vi "Format CSV.vi"(8 "error in (no error)":errorcluster, 9 "delimiter":string=",", 10 "CSV File Input":path, 11 "Original CSV Format":enum16{"Format A", "Format B"}(ring)) -> (0 "error out":errorcluster, 1 "Parcel Length":i32[](array[numeric]), 2 "All Terminal Data":T1(array[cluster]))   [LabVIEW 2017] (continued)
"40:47.0", "40:47.1", "40:47.1", "40:47.1", "40:47.2", "40:47.2", "40:47.2", "40:47.3", "40:47.3", "40:47.3", "40:47.4", "40:47.4", "40:47.4", "40:47.5", "40:47.5", "40:47.5", "40:47.6", "40:47.6", "40:47.6", "40:47.7", "40:47.7", "40:47.7", "40:47.8", "40:47.8", "40:47.8", "40:47.9", "40:47.9", "40:47.9", "40:48.0", "40:48.0", "40:48.0", "40:48.1", "40:48.1", "40:48.1", "40:48.2", "40:48.2", "40:48.2", "40:48.3", "40:48.3", "40:48.3", "40:48.4", "40:48.4", "40:48.4", "40:48.5", "40:48.5", "40:48.5", "40:48.6", "40:48.6", "40:48.6", "40:48.7", "40:48.7", "40:48.7", "40:48.8", "40:48.8", "40:48.8", "40:48.9", "40:48.9", "40:48.9", "40:49.0", "40:49.0", "40:49.0", "40:49.1", "40:49.1", "40:49.1", "40:49.2", "40:49.2", "40:49.2", "40:49.3", "40:49.3", "40:49.3", "40:49.4", "40:49.4", "40:49.4", "40:49.5", "40:49.5", "40:49.5", "40:49.6", "40:49.6", "40:49.6", "40:49.7", "40:49.7", "40:49.7", "40:49.8", "40:49.8", "40:49.8", "40:49.9", "40:49.9", "40:49.9", "40:50.0", "40:50.0", "40:50.0", "40:50.1", "40:50.1", "40:50.1", "40:50.2", "40:50.2", "40:50.2", "40:50.3", "40:50.3", "40:50.3", "40:50.4", "40:50.4", "40:50.4", "40:50.5", "40:50.5", "40:50.5", "40:50.6", "40:50.6", "40:50.6", "40:50.7", "40:50.7", "40:50.7", "40:50.8", "40:50.8", "40:50.8", "40:50.9", "40:50.9", "40:50.9", "40:51.0", "40:51.0", "40:51.0", "40:51.1", "40:51.1", "40:51.1", "40:51.2", "40:51.2", "40:51.2", "40:51.3", "40:51.3", "40:51.3", "40:51.4", "40:51.4", "40:51.4", "40:51.5", "40:51.5", "40:51.5", "40:51.6", "40:51.6", "40:51.6", "40:51.7", "40:51.7", "40:51.7", "40:51.8", "40:51.8", "40:51.8", "40:51.9", "40:51.9", "40:51.9", "40:52.0", "40:52.0", "40:52.0", "40:52.1", "40:52.1", "40:52.1", "40:52.2", "40:52.2", "40:52.2", "40:52.3", "40:52.3", "40:52.3", "40:52.4", "40:52.4", "40:52.4", "40:52.5", "40:52.5", "40:52.5", "40:52.6", "40:52.6", "40:52.6", "40:52.7", "40:52.7", "40:52.7", "40:52.8", "40:52.8", "40:52.8", "40:52.9", "40:52.9", "40:52.9", "40:53.0", "40:53.0", "40:53.0", "40:53.1", "40:53.1", "40:53.1", "40:53.2", "40:53.2", "40:53.2", "40:53.3", "40:53.3", "40:53.3", "40:53.4", "40:53.4", "40:53.4", "40:53.5", "40:53.5", "40:53.5", "40:53.6", "40:53.6", "40:53.6", "40:53.7", "40:53.7", "40:53.7", "40:53.8", "40:53.8", "40:53.8", "40:53.9", "40:53.9", "40:53.9", "40:54.0", "40:54.0", "40:54.0", "40:54.1", "40:54.1", "40:54.1", "40:54.2", "40:54.2", "40:54.2", "40:54.3", "40:54.3", "40:54.3", "40:54.4", "40:54.4", "40:54.4", "40:54.5", "40:54.5", "40:54.5", "40:54.6", "40:54.6", "40:54.6", "40:54.7", "40:54.7", "40:54.7", "40:54.8", "40:54.8", "40:54.8", "40:54.9", "40:54.9", "40:54.9", "40:55.0", "40:55.0", "40:55.0", "40:55.1", "40:55.1", "40:55.1", "40:55.2", "40:55.2", "40:55.2", "40:55.3", "40:55.3", "40:55.3", "40:55.4", "40:55.4", "40:55.4", "40:55.5", "40:55.5", "40:55.5", "40:55.6", "40:55.6", "40:55.6", "40:55.7", "40:55.7", "40:55.7", "40:55.8", "40:55.8", "40:55.8", "40:55.9", "40:55.9", "40:55.9", "40:56.0", "40:56.0", "40:56.0", "40:56.1", "40:56.1", "40:56.1", "40:56.2", "40:56.2", "40:56.2", "40:56.3", "40:56.3", "40:56.3", "40:56.4", "40:56.4", "40:56.4", "40:56.5", "40:56.5", "40:56.5", "40:56.6", "40:56.6", "40:56.6", "40:56.7", "40:56.7", "40:56.7", "40:56.8", "40:56.8", "40:56.8", "40:56.9", "40:56.9", "40:56.9", "40:57.0", "40:57.0", "40:57.0", "40:57.1", "40:57.1", "40:57.1", "40:57.2", "40:57.2", "40:57.2", "40:57.3", "40:57.3", "40:57.3", "40:57.4", "40:57.4", "40:57.4", "40:57.5", "40:57.5", "40:57.5", "40:57.6", "40:57.6", "40:57.6", "40:57.7", "40:57.7", "40:57.7", "40:57.8", "40:57.8", "40:57.8", "40:57.9", "40:57.9", "40:57.9", "40:58.0", "40:58.0", "40:58.0", "40:58.1", "40:58.1", "40:58.1", "40:58.2", "40:58.2", "40:58.2", "40:58.3", "40:58.3", "40:58.3", "40:58.4", "40:58.4", "40:58.4", "40:58.5", "40:58.5", "40:58.5", "40:58.6", "40:58.6", "40:58.6", "40:58.7", "40:58.7", "40:58.7", "40:58.8", "40:58.8", "40:58.8", "40:58.9", "40:58.9", "40:58.9", "40:59.0", "40:59.0", "40:59.0", "40:59.1", "40:59.1", "40:59.1", "40:59.2", "40:59.2", "40:59.2", "40:59.3", "40:59.3", "40:59.3", "40:59.4", "40:59.4", "40:59.4", "40:59.5", "40:59.5", "40:59.5", "40:59.6", "40:59.6", "40:59.6", "40:59.7", "40:59.7", "40:59.7", "40:59.8", "40:59.8", "40:59.8", "40:59.9", "40:59.9", "40:59.9", "41:00.0", "41:00.0", "41:00.0", "41:00.1", "41:00.1", "41:00.1", "41:00.2", "41:00.2", "41:00.2", "41:00.3", "41:00.3", "41:00.3", "41:00.4", "41:00.4", "41:00.4", "41:00.5", "41:00.5", "41:00.5", "41:00.6", "41:00.6", "41:00.6", "41:00.7", "41:00.7", "41:00.7", "41:00.8", "41:00.8", "41:00.8", "41:00.9", "41:00.9", "41:00.9", "41:01.0", "41:01.0", "41:01.0", "41:01.1", "41:01.1", "41:01.1", "41:01.2", "41:01.2", "41:01.2", "41:01.3", "41:01.3", "41:01.3", "41:01.4", "41:01.4", "41:01.4", "41:01.5", "41:01.5", "41:01.5", "41:01.6", "41:01.6", "41:01.6", "41:01.7", "41:01.7", "41:01.7", "41:01.8", "41:01.8", "41:01.8", "41:01.9", "41:01.9", "41:01.9", "41:02.0", "41:02.0", "41:02.0", "41:02.1", "41:02.1", "41:02.1", "41:02.2", "41:02.2", "41:02.2", "41:02.3", "41:02.3", "41:02.3", "41:02.4", "41:02.4", "41:02.4", "41:02.5", "41:02.5", "41:02.5", "41:02.6", "41:02.6", "41:02.6", "41:02.7", "41:02.7", "41:02.7", "41:02.8", "41:02.8", "41:02.8", "41:02.9", "41:02.9", "41:02.9", "41:03.0", "41:03.0", "41:03.0", "41:03.1", "41:03.1", "41:03.1", "41:03.2", "41:03.2", "41:03.2", "41:03.3", "41:03.3", "41:03.3", "41:03.4", "41:03.4", "41:03.4", "41:03.5", "41:03.5", "41:03.5", "41:03.6", "41:03.6", "41:03.6", "41:03.7", "41:03.7", "41:03.7", "41:03.8", "41:03.8", "41:03.8", "41:03.9", "41:03.9", "41:03.9", "41:04.0", "41:04.0", "41:04.0", "41:04.1", "41:04.1", "41:04.1", "41:04.2", "41:04.2", "41:04.2", "41:04.3", "41:04.3", "41:04.3", "41:04.4", "41:04.4", "41:04.4", "41:04.5", "41:04.5", "41:04.5", "41:04.6", "41:04.6", "41:04.6", "41:04.7", "41:04.7", "41:04.7", "41:04.8", "41:04.8", "41:04.8", "41:04.9", "41:04.9", "41:04.9", "41:05.0", "41:05.0", "41:05.0", "41:05.1", "41:05.1", "41:05.1", "41:05.2", "41:05.2", "41:05.2", "41:05.3", "41:05.3", "41:05.3", "41:05.4", "41:05.4", "41:05.4", "41:05.5", "41:05.5", "41:05.5", "41:05.6", "41:05.6", "41:05.6", "41:05.7", "41:05.7", "41:05.7", "41:05.8", "41:05.8", "41:05.8", "41:05.9", "41:05.9", "41:05.9", "41:06.0", "41:06.0", "41:06.0", "41:06.1", "41:06.1", "41:06.1", "41:06.2", "41:06.2", "41:06.2", "41:06.3", "41:06.3", "41:06.3", "41:06.4", "41:06.4", "41:06.4", "41:06.5", "41:06.5", "41:06.5", "41:06.6", "41:06.6", "41:06.6", "41:06.7", "41:06.7", "41:06.7", "41:06.8", "41:06.8", "41:06.8", "41:06.9", "41:06.9", "41:06.9", "41:07.0", "41:07.0", "41:07.0", "41:07.1", "41:07.1", "41:07.1", "41:07.2", "41:07.2", "41:07.2", "41:07.3", "41:07.3", "41:07.3", "41:07.4", "41:07.4", "41:07.4", "41:07.5", "41:07.5", "41:07.5", "41:07.6", "41:07.6", "41:07.6", "41:07.7", "41:07.7", "41:07.7", "41:07.8", "41:07.8", "41:07.8", "41:07.9", "41:07.9", "41:07.9", "41:08.0", "41:08.0", "41:08.0", "41:08.1", "41:08.1", "41:08.1", "41:08.2", "41:08.2", "41:08.2", "41:08.3", "41:08.3", "41:08.3", "41:08.4", "41:08.4", "41:08.4", "41:08.5", "41:08.5", "41:08.5", "41:08.6", "41:08.6", "41:08.6", "41:08.7", "41:08.7", "41:08.7", "41:08.8", "41:08.8", "41:08.8", "41:08.9", "41:08.9", "41:08.9", "41:09.0", "41:09.0", "41:09.0", "41:09.1", "41:09.1", "41:09.1", "41:09.2", "41:09.2", "41:09.2", "41:09.3", "41:09.3", "41:09.3", "41:09.4", "41:09.4", "41:09.4", "41:09.5", "41:09.5", "41:09.5", "41:09.6", "41:09.6", "41:09.6", "41:09.7", "41:09.7", "41:09.7", "41:09.8", "41:09.8", "41:09.8", "41:09.9", "41:09.9", "41:09.9", "41:10.0", "41:10.0", "41:10.0", "41:10.1", "41:10.1", "41:10.1", "41:10.2", "41:10.2", "41:10.2", "41:10.3", "41:10.3", "41:10.3", "41:10.4", "41:10.4", "41:10.4", "41:10.5", "41:10.5", "41:10.5", "41:10.6", "41:10.6", "41:10.6", "41:10.7", "41:10.7", "41:10.7", "41:10.8", "41:10.8", "41:10.8", "41:10.9", "41:10.9", "41:10.9", "41:11.0", "41:11.0", "41:11.0", "41:11.1", "41:11.1", "41:11.1", "41:11.2", "41:11.2", "41:11.2", "41:11.3", "41:11.3", "41:11.3", "41:11.4", "41:11.4", "41:11.4", "41:11.5", "41:11.5", "41:11.5", "41:11.6", "41:11.6", "41:11.6", "41:11.7", "41:11.7", "41:11.7", "41:11.8", "41:11.8", "41:11.8", "41:11.9", "41:11.9", "41:11.9", "41:12.0", "41:12.0", "41:12.0", "41:12.1", "41:12.1", "41:12.1", "41:12.2", "41:12.2", "41:12.2", "41:12.3", "41:12.3", "41:12.3", "41:12.4", "41:12.4", "41:12.4", "41:12.5", "41:12.5", "41:12.5", "41:12.6", "41:12.6", "41:12.6", "41:12.7", "41:12.7", "41:12.7", "41:12.8", "41:12.8", "41:12.8", "41:12.9", "41:12.9", "41:12.9", "41:13.0", "41:13.0", "41:13.0", "41:13.1", "41:13.1", "41:13.1", "41:13.2", "41:13.2", "41:13.2", "41:13.3", "41:13.3", "41:13.3", "41:13.4", "41:13.4", "41:13.4", "41:13.5", "41:13.5", "41:13.5", "41:13.6", "41:13.6", "41:13.6", "41:13.7", "41:13.7", "41:13.7", "41:13.8", "41:13.8", "41:13.8", "41:13.9", "41:13.9", "41:13.9", "41:14.0", "41:14.0", "41:14.0", "41:14.1", "41:14.1", "41:14.1", "41:14.2", "41:14.2", "41:14.2", "41:14.3", "41:14.3", "41:14.3", "41:14.4", "41:14.4", "41:14.4", "41:14.5", "41:14.5", "41:14.5", "41:14.6", "41:14.6", "41:14.6", "41:14.7", "41:14.7", "41:14.7", "41:14.8", "41:14.8", "41:14.8", "41:14.9", "41:14.9", "41:14.9", "41:15.0", "41:15.0", "41:15.0", "41:15.1", "41:15.1", "41:15.1", "41:15.2", "41:15.2", "41:15.2", "41:15.3", "41:15.3", "41:15.3", "41:15.4", "41:15.4", "41:15.4", "41:15.5", "41:15.5", "41:15.5", "41:15.6", "41:15.6", "41:15.6", "41:15.7", "41:15.7", "41:15.7", "41:15.8", "41:15.8", "41:15.8", "41:15.9", "41:15.9", "41:15.9", "41:16.0", "41:16.0", "41:16.0", "41:16.1", "41:16.1", "41:16.1", "41:16.2", "41:16.2", "41:16.2", "41:16.3", "41:16.3", "41:16.3", "41:16.4", "41:16.4", "41:16.4", "41:16.5", "41:16.5", "41:16.5", "41:16.6", "41:16.6", "41:16.6", "41:16.7", "41:16.7", "41:16.7", "41:16.8", "41:16.8", "41:16.8", "41:16.9", "41:16.9", "41:16.9", "41:17.0", "41:17.0", "41:17.0", "41:17.1", "41:17.1", "41:17.1", "41:17.2", "41:17.2", "41:17.2", "41:17.3", "41:17.3", "41:17.3", "41:17.4", "41:17.4", "41:17.4", "41:17.5", "41:17.5", "41:17.5", "41:17.6", "41:17.6", "41:17.6", "41:17.7", "41:17.7", "41:17.7", "41:17.8", "41:17.8", "41:17.8", "41:17.9", "41:17.9", "41:17.9", "41:18.0", "41:18.0", "41:18.0", "41:18.1", "41:18.1", "41:18.1", "41:18.2", "41:18.2", "41:18.2", "41:18.3", "41:18.3", "41:18.3", "41:18.4", "41:18.4", "41:18.4", "41:18.5", "41:18.5", "41:18.5", "41:18.6", "41:18.6", "41:18.6", "41:18.7", "41:18.7", "41:18.7", "41:18.8", "41:18.8", "41:18.8", "41:18.9", "41:18.9", "41:18.9", "41:19.0", "41:19.0", "41:19.0", "41:19.1", "41:19.1", "41:19.1", "41:19.2", "41:19.2", "41:19.2", "41:19.3", "41:19.3", "41:19.3", "41:19.4", "41:19.4", "41:19.4", "41:19.5", "41:19.5", "41:19.5", "41:19.6", "41:19.6", "41:19.6", "41:19.7", "41:19.7", "41:19.7", "41:19.8", "41:19.8", "41:19.8", "41:19.9", "41:19.9", "41:19.9", "41:20.0", "41:20.0", "41:20.0", "41:20.1", "41:20.1", "41:20.1", "41:20.2", "41:20.2", "41:20.2", "41:20.3", "41:20.3", "41:20.3", "41:20.4", "41:20.4", "41:20.4", "41:20.5", "41:20.5", "41:20.5", "41:20.6", "41:20.6", "41:20.6", "41:20.7", "41:20.7", "41:20.7", "41:20.8", "41:20.8", "41:20.8", "41:20.9", "41:20.9", "41:20.9", "41:21.0", "41:21.0", "41:21.0", "41:21.1", "41:21.1", "41:21.1", "41:21.2", "41:21.2", "41:21.2", "41:21.3", "41:21.3", "41:21.3", "41:21.4", "41:21.4", "41:21.4", "41:21.5", "41:21.5", "41:21.5", "41:21.6", "41:21.6", "41:21.6", "41:21.7", "41:21.7", "41:21.7", "41:21.8", "41:21.8", "41:21.8", "41:21.9", "41:21.9", "41:21.9", "41:22.0", "41:22.0", "41:22.0", "41:22.1", "41:22.1", "41:22.1", "41:22.2", "41:22.2", "41:22.2", "41:22.3", "41:22.3", "41:22.3", "41:22.4", "41:22.4", "41:22.4", "41:22.5", "41:22.5", "41:22.5", "41:22.6", "41:22.6", "41:22.6", "41:22.7", "41:22.7", "41:22.7", "41:22.8", "41:22.8", "41:22.8", "41:22.9", "41:22.9", "41:22.9", "41:23.0", "41:23.0", "41:23.0", "41:23.1", "41:23.1", "41:23.1", "41:23.2", "41:23.2", "41:23.2", "41:23.3", "41:23.3", "41:23.3", "41:23.4", "41:23.4", "41:23.4", "41:23.5", "41:23.5", "41:23.5", "41:23.6", "41:23.6", "41:23.6", "41:23.7", "41:23.7", "41:23.7", "41:23.8", "41:23.8", "41:23.8", "41:23.9", "41:23.9", "41:23.9", "41:24.0", "41:24.0", "41:24.0", "41:24.1", "41:24.1", "41:24.1", "41:24.2", "41:24.2", "41:24.2", "41:24.3", "41:24.3", "41:24.3", "41:24.4", "41:24.4", "41:24.4", "41:24.5", "41:24.5", "41:24.5", "41:24.6", "41:24.6", "41:24.6", "41:24.7", "41:24.7", "41:24.7", "41:24.8", "41:24.8", "41:24.8", "41:24.9", "41:24.9", "41:24.9", "41:25.0", "41:25.0", "41:25.0", "41:25.1", "41:25.1", "41:25.1", "41:25.2", "41:25.2", "41:25.2", "41:25.3", "41:25.3", "41:25.3", "41:25.4", "41:25.4", "41:25.4", "41:25.5", "41:25.5", "41:25.5", "41:25.6", "41:25.6", "41:25.6", "41:25.7", "41:25.7", "41:25.7", "41:25.8", "41:25.8", "41:25.8", "41:25.9", "41:25.9", "41:25.9", "41:26.0", "41:26.0", "41:26.0", "41:26.1", "41:26.1", "41:26.1", "41:26.2", "41:26.2", "41:26.2", "41:26.3", "41:26.3", "41:26.3", "41:26.4", "41:26.4", "41:26.4", "41:26.5", "41:26.5", "41:26.5", "41:26.6", "41:26.6", "41:26.6", "41:26.7", "41:26.7", "41:26.7", "41:26.8", "41:26.8", "41:26.8", "41:26.9", "41:26.9", "41:26.9", "41:27.0", "41:27.0", "41:27.0", "41:27.1", "41:27.1", "41:27.1", "41:27.2", "41:27.2", "41:27.2", "41:27.3", "41:27.3", "41:27.3", "41:27.4", "41:27.4", "41:27.4", "41:27.5", "41:27.5", "41:27.5", "41:27.6", "41:27.6", "41:27.6", "41:27.7", "41:27.7", "41:27.7", "41:27.8", "41:27.8", "41:27.8", "41:27.9", "41:27.9", "41:27.9", "41:28.0", "41:28.0", "41:28.0", "41:28.1", "41:28.1", "41:28.1", "41:28.2", "41:28.2", "41:28.2", "41:28.3", "41:28.3", "41:28.3", "41:28.4", "41:28.4", "41:28.4", "41:28.5", "41:28.5", "41:28.5", "41:28.6", "41:28.6", "41:28.6", "41:28.7", "41:28.7", "41:28.7", "41:28.8", "41:28.8", "41:28.8", "41:28.9", "41:28.9", "41:28.9", "41:29.0", "41:29.0", "41:29.0", "41:29.1", "41:29.1", "41:29.1", "41:29.2", "41:29.2", "41:29.2", "41:29.3", "41:29.3", "41:29.3", "41:29.4", "41:29.4", "41:29.4", "41:29.5", "41:29.5", "41:29.5", "41:29.6", "41:29.6", "41:29.6", "41:29.7", "41:29.7", "41:29.7", "41:29.8", "41:29.8", "41:29.8", "41:29.9", "41:29.9", "41:29.9", "41:30.0", "41:30.0", "41:30.0", "41:30.1", "41:30.1", "41:30.1", "41:30.2", "41:30.2", "41:30.2", "41:30.3", "41:30.3", "41:30.3", "41:30.4", "41:30.4", "41:30.4", "41:30.5", "41:30.5", "41:30.5", "41:30.6", "41:30.6", "41:30.6", "41:30.7", "41:30.7", "41:30.7", "41:30.8", "41:30.8", "41:30.8", "41:30.9", "41:30.9", "41:30.9", "41:31.0", "41:31.0", "41:31.0", "41:31.1", "41:31.1", "41:31.1", "41:31.2", "41:31.2", "41:31.2", "41:31.3", "41:31.3", "41:31.3", "41:31.4", "41:31.4", "41:31.4", "41:31.5", "41:31.5", "41:31.5", "41:31.6", "41:31.6", "41:31.6", "41:31.7", "41:31.7", "41:31.7", "41:31.8", "41:31.8", "41:31.8", "41:31.9", "41:31.9", "41:31.9", "41:32.0", "41:32.0", "41:32.0", "41:32.1", "41:32.1", "41:32.1", "41:32.2", "41:32.2", "41:32.2", "41:32.3", "41:32.3", "41:32.3", "41:32.4", "41:32.4", "41:32.4", "41:32.5", "41:32.5", "41:32.5", "41:32.6", "41:32.6", "41:32.6", "41:32.7", "41:32.7", "41:32.7", "41:32.8", "41:32.8", "41:32.8", "41:32.9", "41:32.9", "41:32.9", "41:33.0", "41:33.0", "41:33.0", "41:33.1", "41:33.1", "41:33.1", "41:33.2", "41:33.2", "41:33.2", "41:33.3", "41:33.3", "41:33.3", "41:33.4", "41:33.4", "41:33.4", "41:33.5", "41:33.5", "41:33.5", "41:33.6", "41:33.6", "41:33.6", "41:33.7", "41:33.7", "41:33.7", "41:33.8", "41:33.8", "41:33.8", "41:33.9", "41:33.9", "41:33.9", "41:34.0", "41:34.0", "41:34.0", "41:34.1", "41:34.1", "41:34.1", "41:34.2", "41:34.2", "41:34.2", "41:34.3", "41:34.3", "41:34.3", "41:34.4", "41:34.4", "41:34.4", "41:34.5", "41:34.5", "41:34.5", "41:34.6", "41:34.6", "41:34.6", "41:34.7", "41:34.7", "41:34.7", "41:34.8", "41:34.8", "41:34.8", "41:34.9", "41:34.9", "41:34.9", "41:35.0", "41:35.0", "41:35.0", "41:35.1", "41:35.1", "41:35.1", "41:35.2", "41:35.2", "41:35.2", "41:35.3", "41:35.3", "41:35.3", "41:35.4", "41:35.4", "41:35.4", "41:35.5", "41:35.5", "41:35.5", "41:35.6", "41:35.6", "41:35.6", "41:35.7", "41:35.7", "41:35.7", "41:35.8", "41:35.8", "41:35.8", "41:35.9", "41:35.9", "41:35.9", "41:36.0", "41:36.0", "41:36.0", "41:36.1", "41:36.1", "41:36.1", "41:36.2", "41:36.2", "41:36.2", "41:36.3", "41:36.3", "41:36.3", "41:36.4", "41:36.4", "41:36.4", "41:36.5", "41:36.5", "41:36.5", "41:36.6", "41:36.6", "41:36.6", "41:36.7", "41:36.7", "41:36.7", "41:36.8", "41:36.8", "41:36.8", "41:36.9", "41:36.9", "41:36.9", "41:37.0", "41:37.0", "41:37.0", "41:37.1", "41:37.1", "41:37.1", "41:37.2", "41:37.2", "41:37.2", "41:37.3", "41:37.3", "41:37.3", "41:37.4", "41:37.4", "41:37.4", "41:37.5", "41:37.5", "41:37.5", "41:37.6", "41:37.6", "41:37.6", "41:37.7", "41:37.7", "41:37.7", "41:37.8", "41:37.8", "41:37.8", "41:37.9", "41:37.9", "41:37.9", "41:38.0", "41:38.0", "41:38.0", "41:38.1", "41:38.1", "41:38.1", "41:38.2", "41:38.2", "41:38.2", "41:38.3", "41:38.3", "41:38.3", "41:38.4", "41:38.4", "41:38.4", "41:38.5", "41:38.5", "41:38.5", "41:38.6", "41:38.6", "41:38.6", "41:38.7", "41:38.7", "41:38.7", "41:38.8", "41:38.8", "41:38.8", "41:38.9", "41:38.9", "41:38.9", "41:39.0", "41:39.0", "41:39.0", "41:39.1", "41:39.1", "41:39.1", "41:39.2", "41:39.2", "41:39.2", "41:39.3", "41:39.3", "41:39.3", "41:39.4", "41:39.4", "41:39.4", "41:39.5", "41:39.5", "41:39.5", "41:39.6", "41:39.6", "41:39.6", "41:39.7", "41:39.7", "41:39.7", "41:39.8", "41:39.8", "41:39.8", "41:39.9", "41:39.9", "41:39.9", "41:40.0", "41:40.0", "41:40.0", "41:40.1", "41:40.1", "41:40.1", "41:40.2", "41:40.2", "41:40.2", "41:40.3", "41:40.3", "41:40.3", "41:40.4", "41:40.4", "41:40.4", "41:40.5", "41:40.5", "41:40.5", "41:40.6", "41:40.6", "41:40.6", "41:40.7", "41:40.7", "41:40.7", "41:40.8", "41:40.8", "41:40.8", "41:40.9", "41:40.9", "41:40.9", "41:41.0", "41:41.0", "41:41.0", "41:41.1", "41:41.1", "41:41.1", "41:41.2", "41:41.2", "41:41.2", "41:41.3", "41:41.3", "41:41.3", "41:41.4", "41:41.4", "41:41.4", "41:41.5", "41:41.5", "41:41.5", "41:41.6", "41:41.6", "41:41.6", "41:41.7", "41:41.7", "41:41.7", "41:41.8", "41:41.8", "41:41.8", "41:41.9", "41:41.9", "41:41.9", "41:42.0", "41:42.0", "41:42.0", "41:42.1", "41:42.1", "41:42.1", "41:42.2", "41:42.2", "41:42.2", "41:42.3", "41:42.3", "41:42.3", "41:42.4", "41:42.4", "41:42.4", "41:42.5", "41:42.5", "41:42.5", "41:42.6", "41:42.6", "41:42.6", "41:42.7", "41:42.7", "41:42.7", "41:42.8", "41:42.8", "41:42.8", "41:42.9", "41:42.9", "41:42.9", "41:43.0", "41:43.0", "41:43.0", "41:43.1", "41:43.1", "41:43.1", "41:43.2", "41:43.2", "41:43.2", "41:43.3", "41:43.3", "41:43.3", "41:43.4", "41:43.4", "41:43.4", "41:43.5", "41:43.5", "41:43.5", "41:43.6", "41:43.6", "41:43.6", "41:43.7", "41:43.7", "41:43.7", "41:43.8", "41:43.8", "41:43.8", "41:43.9", "41:43.9", "41:43.9", "41:44.0", "41:44.0", "41:44.0", "41:44.1", "41:44.1", "41:44.1", "41:44.2", "41:44.2", "41:44.2", "41:44.3", "41:44.3", "41:44.3", "41:44.4", "41:44.4", "41:44.4", "41:44.5", "41:44.5", "41:44.5", "41:44.6", "41:44.6", "41:44.6", "41:44.7", "41:44.7", "41:44.7", "41:44.8", "41:44.8", "41:44.8", "41:44.9", "41:44.9", "41:44.9", "41:45.0", "41:45.0", "41:45.0", "41:45.1", "41:45.1", "41:45.1", "41:45.2", "41:45.2", "41:45.2", "41:45.3", "41:45.3", "41:45.3", "41:45.4", "41:45.4", "41:45.4", "41:45.5", "41:45.5", "41:45.5", "41:45.6", "41:45.6", "41:45.6", "41:45.7", "41:45.7", "41:45.7", "41:45.8", "41:45.8", "41:45.8", "41:45.9", "41:45.9", "41:45.9", "41:46.0", "41:46.0", "41:46.0", "41:46.1", "41:46.1", "41:46.1", "41:46.2", "41:46.2", "41:46.2", "41:46.3", "41:46.3", "41:46.3", "41:46.4", "41:46.4", "41:46.4", "41:46.5", "41:46.5", "41:46.5", "41:46.6", "41:46.6", "41:46.6", "41:46.7", "41:46.7", "41:46.7", "41:46.8", "41:46.8", "41:46.8", "41:46.9", "41:46.9", "41:46.9", "41:47.0", "41:47.0", "41:47.0", "41:47.1", "41:47.1", "41:47.1", "41:47.2", "41:47.2", "41:47.2", "41:47.3", "41:47.3", "41:47.3", "41:47.4", "41:47.4", "41:47.4", "41:47.5", "41:47.5", "41:47.5", "41:47.6", "41:47.6", "41:47.6", "41:47.7", "41:47.7", "41:47.7", "41:47.8", "41:47.8", "41:47.8", "41:47.9", "41:47.9", "41:47.9", "41:48.0", "41:48.0", "41:48.0", "41:48.1", "41:48.1", "41:48.1", "41:48.2", "41:48.2", "41:48.2", "41:48.3", "41:48.3", "41:48.3", "41:48.4", "41:48.4", "41:48.4", "41:48.5", "41:48.5", "41:48.5", "41:48.6", "41:48.6", "41:48.6", "41:48.7", "41:48.7", "41:48.7", "41:48.8", "41:48.8", "41:48.8", "41:48.9", "41:48.9", "41:48.9", "41:49.0", "41:49.0", "41:49.0", "41:49.1", "41:49.1", "41:49.1", "41:49.2", "41:49.2", "41:49.2", "41:49.3", "41:49.3", "41:49.3", "41:49.4", "41:49.4", "41:49.4", "41:49.5", "41:49.5", "41:49.5", "41:49.6", "41:49.6", "41:49.6", "41:49.7", "41:49.7", "41:49.7", "41:49.8", "41:49.8", "41:49.8", "41:49.9", "41:49.9", "41:49.9", "41:50.0", "41:50.0", "41:50.0", "41:50.1", "41:50.1", "41:50.1", "41:50.2", "41:50.2", "41:50.2", "41:50.3", "41:50.3", "41:50.3", "41:50.4", "41:50.4", "41:50.4", "41:50.5", "41:50.5", "41:50.5", "41:50.6", "41:50.6", "41:50.6", "41:50.7", "41:50.7", "41:50.7", "41:50.8", "41:50.8", "41:50.8", "41:50.9", "41:50.9", "41:50.9", "41:51.0", "41:51.0", "41:51.0", "41:51.1", "41:51.1", "41:51.1", "41:51.2", "41:51.2", "41:51.2", "41:51.3", "41:51.3", "41:51.3", "41:51.4", "41:51.4", "41:51.4", "41:51.5", "41:51.5", "41:51.5", "41:51.6", "41:51.6", "41:51.6", "41:51.7", "41:51.7", "41:51.7", "41:51.8", "41:51.8", "41:51.8", "41:51.9", "41:51.9", "41:51.9", "41:52.0", "41:52.0", "41:52.0", "41:52.1", "41:52.1", "41:52.1", "41:52.2", "41:52.2", "41:52.2", "41:52.3", "41:52.3", "41:52.3", "41:52.4", "41:52.4", "41:52.4", "41:52.5", "41:52.5", "41:52.5", "41:52.6", "41:52.6", "41:52.6", "41:52.7", "41:52.7", "41:52.7", "41:52.8", "41:52.8", "41:52.8", "41:52.9", "41:52.9", "41:52.9", "41:53.0", "41:53.0", "41:53.0", "41:53.1", "41:53.1", "41:53.1", "41:53.2", "41:53.2", "41:53.2", "41:53.3", "41:53.3", "41:53.3", "41:53.4", "41:53.4", "41:53.4", "41:53.5", "41:53.5", "41:53.5", "41:53.6", "41:53.6", "41:53.6", "41:53.7", "41:53.7", "41:53.7", "41:53.8", "41:53.8", "41:53.8", "41:53.9", "41:53.9", "41:53.9", "41:54.0", "41:54.0", "41:54.0", "41:54.1", "41:54.1", "41:54.1", "41:54.2", "41:54.2", "41:54.2", "41:54.3", "41:54.3", "41:54.3", "41:54.4", "41:54.4", "41:54.4", "41:54.5", "41:54.5", "41:54.5", "41:54.6", "41:54.6", "41:54.6", "41:54.7", "41:54.7", "41:54.7", "41:54.8", "41:54.8", "41:54.8", "41:54.9", "41:54.9", "41:54.9", "41:55.0", "41:55.0", "41:55.0", "41:55.1", "41:55.1", "41:55.1", "41:55.2", "41:55.2", "41:55.2", "41:55.3", "41:55.3", "41:55.3", "41:55.4", "41:55.4", "41:55.4", "41:55.5", "41:55.5", "41:55.5", "41:55.6", "41:55.6", "41:55.6", "41:55.7", "41:55.7", "41:55.7", "41:55.8", "41:55.8", "41:55.8", "41:55.9", "41:55.9", "41:55.9", "41:56.0", "41:56.0", "41:56.0", "41:56.1", "41:56.1", "41:56.1", "41:56.2", "41:56.2", "41:56.2", "41:56.3", "41:56.3", "41:56.3", "41:56.4", "41:56.4", "41:56.4", "41:56.5", "41:56.5", "41:56.5", "41:56.6", "41:56.6", "41:56.6", "41:56.7", "41:56.7", "41:56.7", "41:56.8", "41:56.8", "41:56.8", "41:56.9", "41:56.9", "41:56.9", "41:57.0", "41:57.0", "41:57.0", "41:57.1", "41:57.1", "41:57.1", "41:57.2", "41:57.2", "41:57.2", "41:57.3", "41:57.3", "41:57.3", "41:57.4", "41:57.4", "41:57.4", "41:57.5", "41:57.5", "41:57.5", "41:57.6", "41:57.6", "41:57.6", "41:57.7", "41:57.7", "41:57.7", "41:57.8", "41:57.8", "41:57.8", "41:57.9", "41:57.9", "41:57.9", "41:58.0", "41:58.0", "41:58.0", "41:58.1", "41:58.1", "41:58.1", "41:58.2", "41:58.2", "41:58.2", "41:58.3", "41:58.3", "41:58.3", "41:58.4", "41:58.4", "41:58.4", "41:58.5", "41:58.5", "41:58.5", "41:58.6", "41:58.6", "41:58.6", "41:58.7", "41:58.7", "41:58.7", "41:58.8", "41:58.8", "41:58.8", "41:58.9", "41:58.9", "41:58.9", "41:59.0", "41:59.0", "41:59.0", "41:59.1", "41:59.1", "41:59.1", "41:59.2", "41:59.2", "41:59.2", "41:59.3", "41:59.3", "41:59.3", "41:59.4", "41:59.4", "41:59.4", "41:59.5", "41:59.5", "41:59.5", "41:59.6", "41:59.6", "41:59.6", "41:59.7", "41:59.7", "41:59.7", "41:59.8", "41:59.8", "41:59.8", "41:59.9", "41:59.9", "41:59.9", "42:00.0", "42:00.0", "42:00.0", "42:00.1", "42:00.1", "42:00.1", "42:00.2", "42:00.2", "42:00.2", "42:00.3", "42:00.3", "42:00.3", "42:00.4", "42:00.4", "42:00.4", "42:00.5", "42:00.5", "42:00.5", "42:00.6", "42:00.6", "42:00.6", "42:00.7", "42:00.7", "42:00.7", "42:00.8", "42:00.8", "42:00.8", "42:00.9", "42:00.9", "42:00.9", "42:01.0", "42:01.0", "42:01.0", "42:01.1", "42:01.1", "42:01.1", "42:01.2", "42:01.2", "42:01.2", "42:01.3", "42:01.3", "42:01.3", "42:01.4", "42:01.4", "42:01.4", "42:01.5", "42:01.5", "42:01.5", "42:01.6", "42:01.6", "42:01.6", "42:01.7", "42:01.7", "42:01.7", "42:01.8", "42:01.8", "42:01.8", "42:01.9", "42:01.9", "42:01.9", "42:02.0", "42:02.0", "42:02.0", "42:02.1", "42:02.1", "42:02.1", "42:02.2", "42:02.2", "42:02.2", "42:02.3", "42:02.3", "42:02.3", "42:02.4", "42:02.4", "42:02.4", "42:02.5", "42:02.5", "42:02.5", "42:02.6", "42:02.6", "42:02.6", "42:02.7", "42:02.7", "42:02.7", "42:02.8", "42:02.8", "42:02.8", "42:02.9", "42:02.9", "42:02.9", "42:03.0", "42:03.0", "42:03.0", "42:03.1", "42:03.1", "42:03.1", "42:03.2", "42:03.2", "42:03.2", "42:03.3", "42:03.3", "42:03.3", "42:03.4", "42:03.4", "42:03.4", "42:03.5", "42:03.5", "42:03.5", "42:03.6", "42:03.6", "42:03.6", "42:03.7", "42:03.7", "42:03.7", "42:03.8", "42:03.8", "42:03.8", "42:03.9", "42:03.9", "42:03.9", "42:04.0", "42:04.0", "42:04.0", "42:04.1", "42:04.1", "42:04.1", "42:04.2", "42:04.2", "42:04.2", "42:04.3", "42:04.3", "42:04.3", "42:04.4", "42:04.4", "42:04.4", "42:04.5", "42:04.5", "42:04.5", "42:04.6", "42:04.6", "42:04.6", "42:04.7", "42:04.7", "42:04.7", "42:04.8", "42:04.8", "42:04.8", "42:04.9", "42:04.9", "42:04.9", "42:05.0", "42:05.0", "42:05.0", "42:05.1", "42:05.1", "42:05.1", "42:05.2", "42:05.2", "42:05.2", "42:05.3", "42:05.3", "42:05.3", "42:05.4", "42:05.4", "42:05.4", "42:05.5", "42:05.5", "42:05.5", "42:05.6", "42:05.6", "42:05.6", "42:05.7", "42:05.7", "42:05.7", "42:05.8", "42:05.8", "42:05.8", "42:05.9", "42:05.9", "42:05.9", "42:06.0", "42:06.0", "42:06.0", "42:06.1", "42:06.1", "42:06.1", "42:06.2", "42:06.2", "42:06.2", "42:06.3", "42:06.3", "42:06.3", "42:06.4", "42:06.4", "42:06.4", "42:06.5", "42:06.5", "42:06.5", "42:06.6", "42:06.6", "42:06.6", "42:06.7", "42:06.7", "42:06.7", "42:06.8", "42:06.8", "42:06.8", "42:06.9", "42:06.9", "42:06.9", "42:07.0", "42:07.0", "42:07.0", "42:07.1", "42:07.1", "42:07.1", "42:07.2", "42:07.2", "42:07.2", "42:07.3", "42:07.3", "42:07.3", "42:07.4", "42:07.4", "42:07.4", "42:07.5", "42:07.5", "42:07.5", "42:07.6", "42:07.6", "42:07.6", "42:07.7", "42:07.7", "42:07.7", "42:07.8", "42:07.8", "42:07.8", "42:07.9", "42:07.9", "42:07.9", "42:08.0", "42:08.0", "42:08.0", "42:08.1", "42:08.1", "42:08.1", "42:08.2", "42:08.2", "42:08.2", "42:08.3", "42:08.3", "42:08.3", "42:08.4", "42:08.4", "42:08.4", "42:08.5", "42:08.5", "42:08.5", "42:08.6", "42:08.6", "42:08.6", "42:08.7", "42:08.7", "42:08.7", "42:08.8", "42:08.8", "42:08.8", "42:08.9", "42:08.9", "42:08.9", "42:09.0", "42:09.0", "42:09.0", "42:09.1", "42:09.1", "42:09.1", "42:09.2", "42:09.2", "42:09.2", "42:09.3", "42:09.3", "42:09.3", "42:09.4", "42:09.4", "42:09.4", "42:09.5", "42:09.5", "42:09.5", "42:09.6", "42:09.6", "42:09.6", "42:09.7", "42:09.7", "42:09.7", "42:09.8", "42:09.8", "42:09.8", "42:09.9", "42:09.9", "42:09.9", "42:10.0", "42:10.0", "42:10.0", "42:10.1", "42:10.1", "42:10.1", "42:10.2", "42:10.2", "42:10.2", "42:10.3", "42:10.3", "42:10.3", "42:10.4", "42:10.4", "42:10.4", "42:10.5", "42:10.5", "42:10.5", "42:10.6", "42:10.6", "42:10.6", "42:10.7", "42:10.7", "42:10.7", "42:10.8", "42:10.8", "42:10.8", "42:10.9", "42:10.9", "42:10.9", "42:11.0", "42:11.0", "42:11.0", "42:11.1", "42:11.1", "42:11.1", "42:11.2", "42:11.2", "42:11.2", "42:11.3", "42:11.3", "42:11.3", "42:11.4", "42:11.4", "42:11.4", "42:11.5", "42:11.5", "42:11.5", "42:11.6", "42:11.6", "42:11.6", "42:11.7", "42:11.7", "42:11.7", "42:11.8", "42:11.8", "42:11.8", "42:11.9", "42:11.9", "42:11.9", "42:12.0", "42:12.0", "42:12.0", "42:12.1", "42:12.1", "42:12.1", "42:12.2", "42:12.2", "42:12.2", "42:12.3", "42:12.3", "42:12.3", "42:12.4", "42:12.4", "42:12.4", "42:12.5", "42:12.5", "42:12.5", "42:12.6", "42:12.6", "42:12.6", "42:12.7", "42:12.7", "42:12.7", "42:12.8", "42:12.8", "42:12.8", "42:12.9", "42:12.9", "42:12.9", "42:13.0", "42:13.0", "42:13.0", "42:13.1", "42:13.1", "42:13.1", "42:13.2", "42:13.2", "42:13.2", "42:13.3", "42:13.3", "42:13.3", "42:13.4", "42:13.4", "42:13.4", "42:13.5", "42:13.5", "42:13.5", "42:13.6", "42:13.6", "42:13.6", "42:13.7", "42:13.7", "42:13.7", "42:13.8", "42:13.8", "42:13.8", "42:13.9", "42:13.9", "42:13.9", "42:14.0", "42:14.0", "42:14.0", "42:14.1", "42:14.1", "42:14.1", "42:14.2", "42:14.2", "42:14.2", "42:14.3", "42:14.3", "42:14.3", "42:14.4", "42:14.4", "42:14.4", "42:14.5", "42:14.5", "42:14.5", "42:14.6", "42:14.6", "42:14.6", "42:14.7", "42:14.7", "42:14.7", "42:14.8", "42:14.8", "42:14.8", "42:14.9", "42:14.9", "42:14.9", "42:15.0", "42:15.0", "42:15.0", "42:15.1", "42:15.1", "42:15.1", "42:15.2", "42:15.2", "42:15.2", "42:15.3", "42:15.3", "42:15.3", "42:15.4", "42:15.4", "42:15.4", "42:15.5", "42:15.5", "42:15.5", "42:15.6", "42:15.6", "42:15.6", "42:15.7", "42:15.7", "42:15.7", "42:15.8", "42:15.8", "42:15.8", "42:15.9", "42:15.9", "42:15.9", "42:16.0", "42:16.0", "42:16.0", "42:16.1", "42:16.1", "42:16.1", "42:16.2", "42:16.2", "42:16.2", "42:16.3", "42:16.3", "42:16.3", "42:16.4", "42:16.4", "42:16.4", "42:16.5", "42:16.5", "42:16.5", "42:16.6", "42:16.6", "42:16.6", "42:16.7", "42:16.7", "42:16.7", "42:16.8", "42:16.8", "42:16.8", "42:16.9", "42:16.9", "42:16.9", "42:17.0", "42:17.0", "42:17.0", "42:17.1", "42:17.1", "42:17.1", "42:17.2", "42:17.2", "42:17.2", "42:17.3", "42:17.3", "42:17.3", "42:17.4", "42:17.4", "42:17.4", "42:17.5", "42:17.5", "42:17.5", "42:17.6", "42:17.6", "42:17.6", "42:17.7", "42:17.7", "42:17.7", "42:17.8", "42:17.8", "42:17.8", "42:17.9", "42:17.9", "42:17.9", "42:18.0", "42:18.0", "42:18.0", "42:18.1", "42:18.1", "42:18.1", "42:18.2", "42:18.2", "42:18.2", "42:18.3", "42:18.3", "42:18.3", "42:18.4", "42:18.4", "42:18.4", "42:18.5", "42:18.5", "42:18.5", "42:18.6", "42:18.6", "42:18.6", "42:18.7", "42:18.7", "42:18.7", "42:18.8", "42:18.8", "42:18.8", "42:18.9", "42:18.9", "42:18.9", "42:19.0", "42:19.0", "42:19.0", "42:19.1", "42:19.1", "42:19.1", "42:19.2", "42:19.2", "42:19.2", "42:19.3", "42:19.3", "42:19.3", "42:19.4", "42:19.4", "42:19.4", "42:19.5", "42:19.5", "42:19.5", "42:19.6", "42:19.6", "42:19.6", "42:19.7", "42:19.7", "42:19.7", "42:19.8", "42:19.8", "42:19.8", "42:19.9", "42:19.9", "42:19.9", "42:20.0", "42:20.0", "42:20.0", "42:20.1", "42:20.1", "42:20.1", "42:20.2", "42:20.2", "42:20.2", "42:20.3", "42:20.3", "42:20.3", "42:20.4", "42:20.4", "42:20.4", "42:20.5", "42:20.5", "42:20.5", "42:20.6", "42:20.6", "42:20.6", "42:20.7", "42:20.7", "42:20.7", "42:20.8", "42:20.8", "42:20.8", "42:20.9", "42:20.9", "42:20.9", "42:21.0", "42:21.0", "42:21.0", "42:21.1", "42:21.1", "42:21.1", "42:21.2", "42:21.2", "42:21.2", "42:21.3", "42:21.3", "42:21.3", "42:21.4", "42:21.4", "42:21.4", "42:21.5", "42:21.5", "42:21.5", "42:21.6", "42:21.6", "42:21.6", "42:21.7", "42:21.7", "42:21.7", "42:21.8", "42:21.8", "42:21.8", "42:21.9", "42:21.9", "42:21.9", "42:22.0", "42:22.0", "42:22.0", "42:22.1", "42:22.1", "42:22.1", "42:22.2", "42:22.2", "42:22.2", "42:22.3", "42:22.3", "42:22.3", "42:22.4", "42:22.4", "42:22.4", "42:22.5", "42:22.5", "42:22.5", "42:22.6", "42:22.6", "42:22.6", "42:22.7", "42:22.7", "42:22.7", "42:22.8", "42:22.8", "42:22.8", "42:22.9", "42:22.9", "42:22.9", "42:23.0", "42:23.0", "42:23.0", "42:23.1", "42:23.1", "42:23.1", "42:23.2", "42:23.2", "42:23.2", "42:23.3", "42:23.3", "42:23.3", "42:23.4", "42:23.4", "42:23.4", "42:23.5", "42:23.5", "42:23.5", "42:23.6", "42:23.6", "42:23.6", "42:23.7", "42:23.7", "42:23.7", "42:23.8", "42:23.8", "42:23.8", "42:23.9", "42:23.9", "42:23.9", "42:24.0", "42:24.0", "42:24.0", "42:24.1", "42:24.1", "42:24.1", "42:24.2", "42:24.2", "42:24.2", "42:24.3", "42:24.3", "42:24.3", "42:24.4", "42:24.4", "42:24.4", "42:24.5", "42:24.5", "42:24.5", "42:24.6", "42:24.6", "42:24.6", "42:24.7", "42:24.7", "42:24.7", "42:24.8", "42:24.8", "42:24.8", "42:24.9", "42:24.9", "42:24.9", "42:25.0", "42:25.0", "42:25.0", "42:25.1", "42:25.1", "42:25.1", "42:25.2", "42:25.2", "42:25.2", "42:25.3", "42:25.3", "42:25.3", "42:25.4", "42:25.4", "42:25.4", "42:25.5", "42:25.5", "42:25.5", "42:25.6", "42:25.6", "42:25.6", "42:25.7", "42:25.7", "42:25.7", "42:25.8", "42:25.8", "42:25.8", "42:25.9", "42:25.9", "42:25.9", "42:26.0", "42:26.0", "42:26.0", "42:26.1", "42:26.1", "42:26.1", "42:26.2", "42:26.2", "42:26.2", "42:26.3", "42:26.3", "42:26.3", "42:26.4", "42:26.4", "42:26.4", "42:26.5", "42:26.5", "42:26.5", "42:26.6", "42:26.6", "42:26.6", "42:26.7", "42:26.7", "42:26.7", "42:26.8", "42:26.8", "42:26.8", "42:26.9", "42:26.9", "42:26.9", "42:27.0", "42:27.0", "42:27.0", "42:27.1", "42:27.1", "42:27.1", "42:27.2", "42:27.2", "42:27.2", "42:27.3", "42:27.3", "42:27.3", "42:27.4", "42:27.4", "42:27.4", "42:27.5", "42:27.5", "42:27.5", "42:27.6", "42:27.6", "42:27.6", "42:27.7", "42:27.7", "42:27.7", "42:27.8", "42:27.8", "42:27.8", "42:27.9", "42:27.9", "42:27.9", "42:28.0", "42:28.0", "42:28.0", "42:28.1", "42:28.1", "42:28.1", "42:28.2", "42:28.2", "42:28.2", "42:28.3", "42:28.3", "42:28.3", "42:28.4", "42:28.4", "42:28.4", "42:28.5", "42:28.5", "42:28.5", "42:28.6", "42:28.6", "42:28.6", "42:28.7", "42:28.7", "42:28.7", "42:28.8", "42:28.8", "42:28.8", "42:28.9", "42:28.9", "42:28.9", "42:29.0", "42:29.0", "42:29.0", "42:29.1", "42:29.1", "42:29.1", "42:29.2", "42:29.2", "42:29.2", "42:29.3", "42:29.3", "42:29.3", "42:29.4", "42:29.4", "42:29.4", "42:29.5", "42:29.5", "42:29.5", "42:29.6", "42:29.6", "42:29.6", "42:29.7", "42:29.7", "42:29.7", "42:29.8", "42:29.8", "42:29.8", "42:29.9", "42:29.9", "42:29.9", "42:30.0", "42:30.0", "42:30.0", "42:30.1", "42:30.1", "42:30.1", "42:30.2", "42:30.2", "42:30.2", "42:30.3", "42:30.3", "42:30.3", "42:30.4", "42:30.4", "42:30.4", "42:30.5", "42:30.5", "42:30.5", "42:30.6", "42:30.6", "42:30.6", "42:30.7", "42:30.7", "42:30.7", "42:30.8", "42:30.8", "42:30.8", "42:30.9", "42:30.9", "42:30.9", "42:31.0", "42:31.0", "42:31.0", "42:31.1", "42:31.1", "42:31.1", "42:31.2", "42:31.2", "42:31.2", "42:31.3", "42:31.3", "42:31.3", "42:31.4", "42:31.4", "42:31.4", "42:31.5", "42:31.5", "42:31.5", "42:31.6", "42:31.6", "42:31.6", "42:31.7", "42:31.7", "42:31.7", "42:31.8", "42:31.8", "42:31.8", "42:31.9", "42:31.9", "42:31.9", "42:32.0", "42:32.0", "42:32.0", "42:32.1", "42:32.1", "42:32.1", "42:32.2", "42:32.2", "42:32.2", "42:32.3", "42:32.3", "42:32.3", "42:32.4", "42:32.4", "42:32.4", "42:32.5", "42:32.5", "42:32.5", "42:32.6", "42:32.6", "42:32.6", "42:32.7", "42:32.7", "42:32.7", "42:32.8", "42:32.8", "42:32.8", "42:32.9", "42:32.9", "42:32.9", "42:33.0", "42:33.0", "42:33.0", "42:33.1", "42:33.1", "42:33.1", "42:33.2", "42:33.2", "42:33.2", "42:33.3", "42:33.3", "42:33.3", "42:33.4", "42:33.4", "42:33.4", "42:33.5", "42:33.5", "42:33.5", "42:33.6", "42:33.6", "42:33.6", "42:33.7", "42:33.7", "42:33.7", "42:33.8", "42:33.8", "42:33.8", "42:33.9", "42:33.9", "42:33.9", "42:34.0", "42:34.0", "42:34.0", "42:34.1", "42:34.1", "42:34.1", "42:34.2", "42:34.2", "42:34.2", "42:34.3", "42:34.3", "42:34.3", "42:34.4", "42:34.4", "42:34.4", "42:34.5", "42:34.5", "42:34.5", "42:34.6", "42:34.6", "42:34.6", "42:34.7", "42:34.7", "42:34.7", "42:34.8", "42:34.8", "42:34.8", "42:34.9", "42:34.9", "42:34.9", "42:35.0", "42:35.0", "42:35.0", "42:35.1", "42:35.1", "42:35.1", "42:35.2", "42:35.2", "42:35.2", "42:35.3", "42:35.3", "42:35.3", "42:35.4", "42:35.4", "42:35.4", "42:35.5", "42:35.5", "42:35.5", "42:35.6", "42:35.6", "42:35.6", "42:35.7", "42:35.7", "42:35.7", "42:35.8", "42:35.8", "42:35.8", "42:35.9", "42:35.9", "42:35.9", "42:36.0", "42:36.0", "42:36.0", "42:36.1", "42:36.1", "42:36.1", "42:36.2", "42:36.2", "42:36.2", "42:36.3", "42:36.3", "42:36.3", "42:36.4", "42:36.4", "42:36.4", "42:36.5", "42:36.5", "42:36.5", "42:36.6", "42:36.6", "42:36.6", "42:36.7", "42:36.7", "42:36.7", "42:36.8", "42:36.8", "42:36.8", "42:36.9", "42:36.9", "42:36.9", "42:37.0", "42:37.0", "42:37.0", "42:37.1", "42:37.1", "42:37.1", "42:37.2", "42:37.2", "42:37.2", "42:37.3", "42:37.3", "42:37.3", "42:37.4", "42:37.4", "42:37.4", "42:37.5", "42:37.5", "42:37.5", "42:37.6", "42:37.6", "42:37.6", "42:37.7", "42:37.7", "42:37.7", "42:37.8", "42:37.8", "42:37.8", "42:37.9", "42:37.9", "42:37.9", "42:38.0", "42:38.0", "42:38.0", "42:38.1", "42:38.1", "42:38.1", "42:38.2", "42:38.2", "42:38.2", "42:38.3", "42:38.3", "42:38.3", "42:38.4", "42:38.4", "42:38.4", "42:38.5", "42:38.5", "42:38.5", "42:38.6", "42:38.6", "42:38.6", "42:38.7", "42:38.7", "42:38.7", "42:38.8", "42:38.8", "42:38.8", "42:38.9", "42:38.9", "42:38.9", "42:39.0", "42:39.0", "42:39.0", "42:39.1", "42:39.1", "42:39.1", "42:39.2", "42:39.2", "42:39.2", "42:39.3", "42:39.3", "42:39.3", "42:39.4", "42:39.4", "42:39.4", "42:39.5", "42:39.5", "42:39.5", "42:39.6", "42:39.6", "42:39.6", "42:39.7", "42:39.7", "42:39.7", "42:39.8", "42:39.8", "42:39.8", "42:39.9", "42:39.9", "42:39.9", "42:40.0", "42:40.0", "42:40.0", "42:40.1", "42:40.1", "42:40.1", "42:40.2", "42:40.2", "42:40.2", "42:40.3", "42:40.3", "42:40.3", "42:40.4", "42:40.4", "42:40.4", "42:40.5", "42:40.5", "42:40.5", "42:40.6", "42:40.6", "42:40.6", "42:40.7", "42:40.7", "42:40.7", "42:40.8", "42:40.8", "42:40.8", "42:40.9", "42:40.9", "42:40.9", "42:41.0", "42:41.0", "42:41.0", "42:41.1", "42:41.1", "42:41.1", "42:41.2", "42:41.2", "42:41.2", "42:41.3", "42:41.3", "42:41.3", "42:41.4", "42:41.4", "42:41.4", "42:41.5", "42:41.5", "42:41.5", "42:41.6", "42:41.6", "42:41.6", "42:41.7", "42:41.7", "42:41.7", "42:41.8", "42:41.8", "42:41.8", "42:41.9", "42:41.9", "42:41.9", "42:42.0", "42:42.0", "42:42.0", "42:42.1", "42:42.1", "42:42.1", "42:42.2", "42:42.2", "42:42.2", "42:42.3", "42:42.3", "42:42.3", "42:42.4", "42:42.4", "42:42.4", "42:42.5", "42:42.5", "42:42.5", "42:42.6", "42:42.6", "42:42.6", "42:42.7", "42:42.7", "42:42.7", "42:42.8", "42:42.8", "42:42.8", "42:42.9", "42:42.9", "42:42.9", "42:43.0", "42:43.0", "42:43.0", "42:43.1", "42:43.1", "42:43.1", "42:43.2", "42:43.2", "42:43.2", "42:43.3", "42:43.3", "42:43.3", "42:43.4", "42:43.4", "42:43.4", "42:43.5", "42:43.5", "42:43.5", "42:43.6", "42:43.6", "42:43.6", "42:43.7", "42:43.7", "42:43.7", "42:43.8", "42:43.8", "42:43.8", "42:43.9", "42:43.9", "42:43.9", "42:44.0", "42:44.0", "42:44.0", "42:44.1", "42:44.1", "42:44.1", "42:44.2", "42:44.2", "42:44.2", "42:44.3", "42:44.3", "42:44.3", "42:44.4", "42:44.4", "42:44.4", "42:44.5", "42:44.5", "42:44.5", "42:44.6", "42:44.6", "42:44.6", "42:44.7", "42:44.7", "42:44.7", "42:44.8", "42:44.8", "42:44.8", "42:44.9", "42:44.9", "42:44.9", "42:45.0", "42:45.0", "42:45.0", "42:45.1", "42:45.1", "42:45.1", "42:45.2", "42:45.2", "42:45.2", "42:45.3", "42:45.3", "42:45.3", "42:45.4", "42:45.4", "42:45.4", "42:45.5", "42:45.5", "42:45.5", "42:45.6", "42:45.6", "42:45.6", "42:45.7", "42:45.7", "42:45.7", "42:45.8", "42:45.8", "42:45.8", "42:45.9", "42:45.9", "42:45.9", "42:46.0", "42:46.0", "42:46.0", "42:46.1", "42:46.1", "42:46.1", "42:46.2", "42:46.2", "42:46.2", "42:46.3", "42:46.3", "42:46.3", "42:46.4", "42:46.4", "42:46.4", "42:46.5", "42:46.5", "42:46.5", "42:46.6", "42:46.6", "42:46.6", "42:46.7", "42:46.7", "42:46.7", "42:46.8", "42:46.8", "42:46.8", "42:46.9", "42:46.9", "42:46.9", "42:47.0", "42:47.0", "42:47.0", "42:47.1", "42:47.1", "42:47.1", "42:47.2", "42:47.2", "42:47.2", "42:47.3", "42:47.3", "42:47.3", "42:47.4", "42:47.4", "42:47.4", "42:47.5", "42:47.5", "42:47.5", "42:47.6", "42:47.6", "42:47.6", "42:47.7", "42:47.7", "42:47.7", "42:47.8", "42:47.8", "42:47.8", "42:47.9", "42:47.9", "42:47.9", "42:48.0", "42:48.0", "42:48.0", "42:48.1", "42:48.1", "42:48.1", "42:48.2", "42:48.2",
